vi "Action Name.vi"(11 "InstallAction in":refnum<class "InstallAction.lvclass">) -> (2 "Action Name":string)   [LabVIEW 2020, in "GPackTools.lvlib" / "InstallAction.lvclass"]
uses:
  InstallAction.lvclass
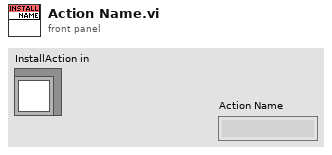
[diagram p1: front panel]
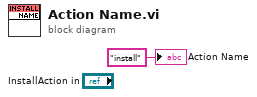
[diagram p0: block diagram]
diagram:
  "Action Name" <- "install" ("Action Name")
